vi "waveform.vi"() -> ()   [LabVIEW 2020]
uses:
  <vilib>/Analysis/NI_AALBase.lvlib
panel:
  in  "Boolean":bool
  in  "Slide":dbl(slide)=1000.0 scale=1.0..100000.0
  in  "dt.ofs":dbl(slide) scale=1.0..10000.0
  in  "pl. wd":dbl(slide) scale=8.0..100.0
  in  "Freq.":dbl(slide) scale=0.0..100.0
  out "Waveform Chart":dbl[](graph)
  out "Waveform Graph":dbl[](graph)
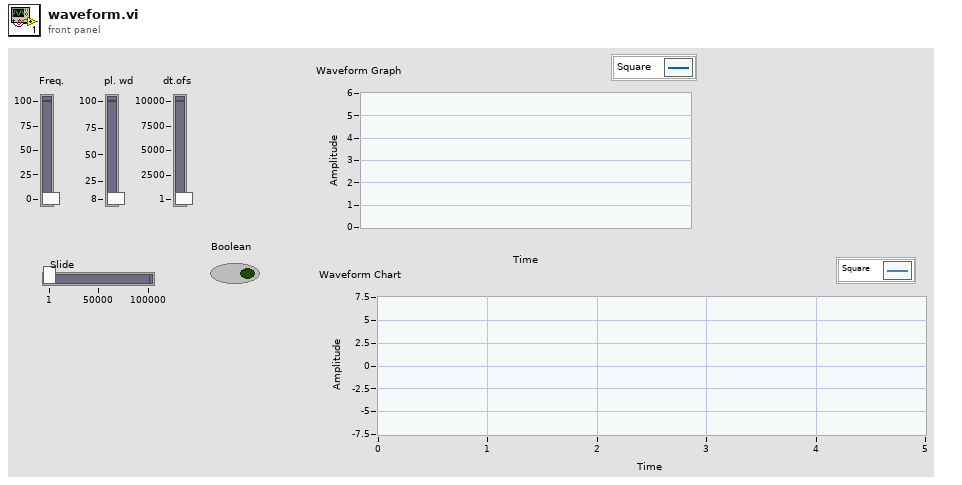
[diagram p1: front panel]
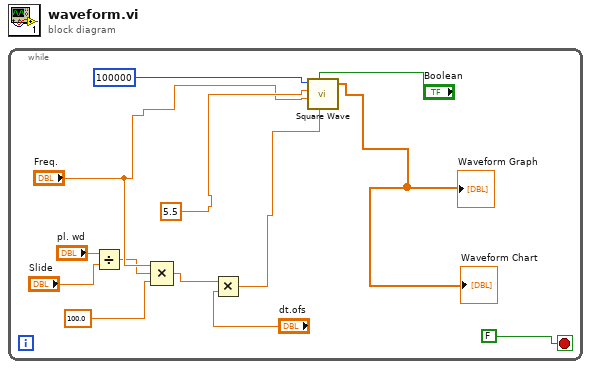
[diagram p0: block diagram]
diagram:
  n1 = while {
    stop <- FALSE stop-if-true
    n2 = Divide(x="pl. wd", y="Slide") -> (x/y=w6:dbl)
    n3 = Compound Arithmetic op=MULTIPLY("Freq.", w6, 100.0) -> (w5:dbl)
    n4 = Multiply(x=w5, y="dt.ofs") -> (x*y=w9:dbl)
    n5 = call <vilib>:"Square Wave.vi"("samples"=100000, "reset phase"="Boolean", "amplitude"=5.5, "frequency"="Freq.", "duty cycle (%)"=w9) -> ("square wave"=→"Waveform Graph" →"Waveform Chart":dbl[])  [unwired: 1 in, 2 out]
  }
